vi "read_weight_files (SubVI).vi"(10 "weight file name":string, 11 "weights path":path) -> (3 "all rows":dbl[][](array[numeric]))   [LabVIEW 2020]
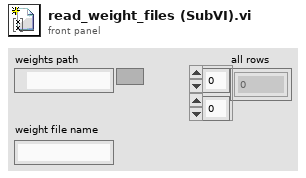
[diagram p1: front panel]
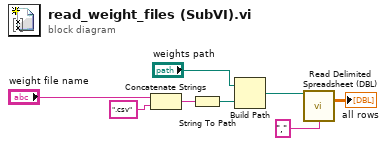
[diagram p0: block diagram]
diagram:
  n1 = Concatenate Strings("weight file name", ".csv") -> (w5:string)
  n2 = String To Path(string=w5) -> (path=w8:path)
  n3 = Build Path(base path="weights path", name or relative path=w8) -> (appended path=w7:path)
  n4 = call <vilib>:"Read Delimited Spreadsheet (DBL).vi"("file path (dialog if empty)"=w7, "delimiter (\\t)"=",") -> ("all rows"=→"all rows":dbl[][])  [unwired: 8 in, 5 out]
